vi "Mono Grating.vi"(8 "error in (no error)":errorcluster, 11 "Mono In":refnum<class "Monochromator.lvclass">) -> (0 "error out":errorcluster, 2 "new Position":i32, 3 "Position":i32)   [LabVIEW 2020, in "Examples.lvlib"]
doc: "This example shows how to get and set the grating position of the mono."
uses:
  Examples.lvlib
  Classes/Mono/Monochromator.lvclass
  0bd624ee-cc67-429d-86ba-aa8b37d700b1.vi
  01530acb-cdb4-4e7f-ad8c-3491b7af0b5d.vi
panel:
  in  "Stop":bool
  # "Connector Pane"
  # "Locals"
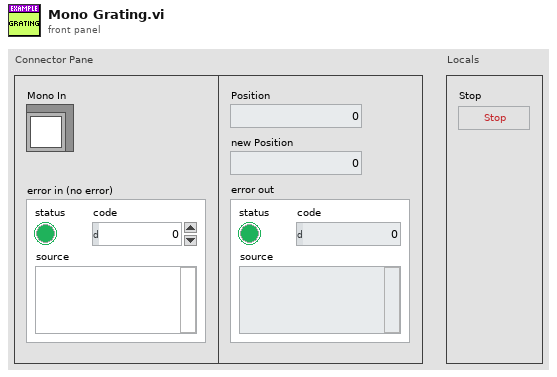
[diagram p1: front panel]
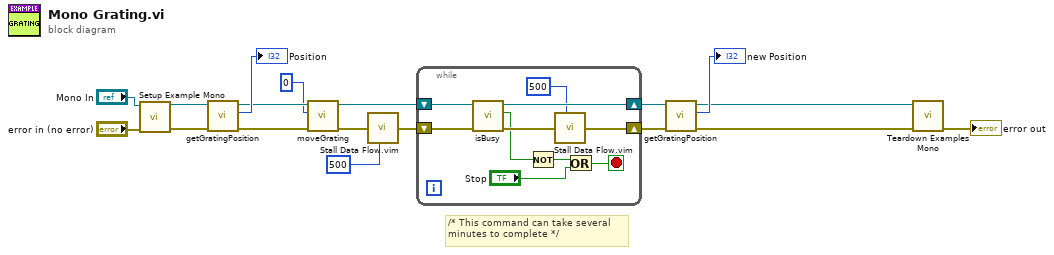
[diagram p0: block diagram]
diagram:
  # "/* This command can take several \nminutes to complete */"
  n1 = call "Setup Example Mono.vi"("error in (no error)"="error in (no error)", "Mono In"="Mono In") -> ("error out"=w14:errorcluster, "Mono Out"=w15:refnum<class "Monochromator.lvclass">)  [unwired: 6 in, 2 out]
  n2 = call "getGratingPosition.vi"("error in (no error)"=w14, "Monochromator in"=w15) -> ("error out"=w10:errorcluster, "Position"=→"Position":i32, "Monochromator out"=w12:refnum<class "Monochromator.lvclass">)  [unwired: 7 in]
  n3 = call "moveGrating.vi"("error in (no error)"=w10, "position"=0, "Monochromator in"=w12) -> ("error out"=w9:errorcluster, "Monochromator out"=w6:refnum<class "Monochromator.lvclass">)  [unwired: 5 in, 2 out]
  n4 = call "Stall Data Flow.vim"("value in"=w9, "milliseconds to wait"=u32 500) -> ("value out"=w8:errorcluster)  [unwired: 1 out]
  n5 = while {
    shift-right: [w24] -> w3
    shift-left: w8 -> [w26]
    shift-right: [w27] -> w4
    shift-left: w6 -> [w25]
    stop <- w21 stop-if-true
    n6 = call "isBusy.vi"("error in (no error)"=w26, "Monochromator in"=w25) -> ("error out"=w28:errorcluster, "mono is busy?"=w22:bool, "Monochromator out"=w27:refnum<class "Monochromator.lvclass">)  [unwired: 7 in]
    n7 = Not(x=w22) -> (.not. x?=w19:bool)
    n8 = call "Stall Data Flow.vim"("value in"=w28, "milliseconds to wait"=u32 500) -> ("value out"=w24:errorcluster)  [unwired: 1 out]
    n9 = Or(x=w19, y="Stop") -> (x .or. y?=w21:bool)
  }
  n10 = call "getGratingPosition.vi"("error in (no error)"=w3, "Monochromator in"=w4) -> ("error out"=w2:errorcluster, "Position"=→"new Position":i32, "Monochromator out"=w1:refnum<class "Monochromator.lvclass">)  [unwired: 7 in]
  n11 = call "Teardown Examples Mono.vi"("error in (no error)"=w2, "Monochromator in"=w1) -> ("error out"=→"error out":errorcluster)  [unwired: 9 in]
